vi "publish-measurements.vi"(5 "hash-format":string="{meas}:%d" caption="hash-format ({meas}:%d)", 7 "ttl":u64=30 caption="ttl (30s)", 8 "error in":errorcluster, 9 "measurement-list":string[](array[string]), 10 "period":u64, 11 "Redis in":refnum<class "Redis.lvclass">) -> (0 "error out":errorcluster, 2 "values":dbl[](array[numeric]), 3 "unix-time":u64)   [LabVIEW 2020, in "reporting-device.lvlib"]
uses:
  reporting-device.lvlib
  <userlib>/Zaphiro/GTools/Redis/Sources/Redis/Redis.lvclass
  <userlib>/Zaphiro/GTools/Redis/Sources/Redis/Redis.lvclass/Redis.ctl
  <userlib>/Zaphiro/GTools/Time/public/convert lv time to unix-scalar__ZGTools.vi
  <userlib>/Zaphiro/GTools/Redis/Sources/Redis/Connection/Send-command.vi
  <userlib>/Zaphiro/GTools/Redis/Sources/Redis/subVIs/LL_collect-response.vi
  <userlib>/Zaphiro/GTools/Time/time__ZGTools.lvlib
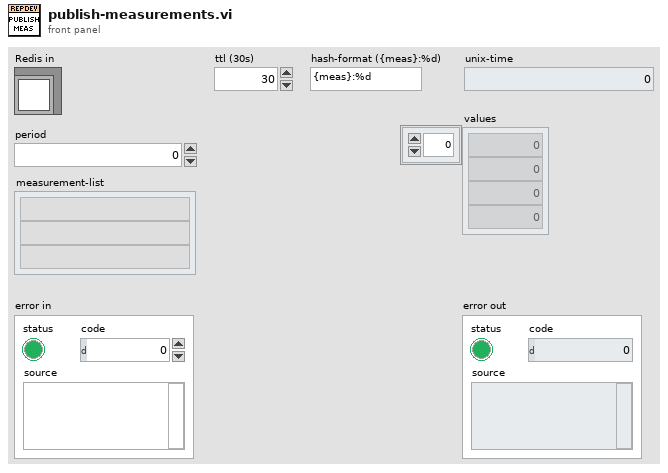
[diagram p1: front panel]
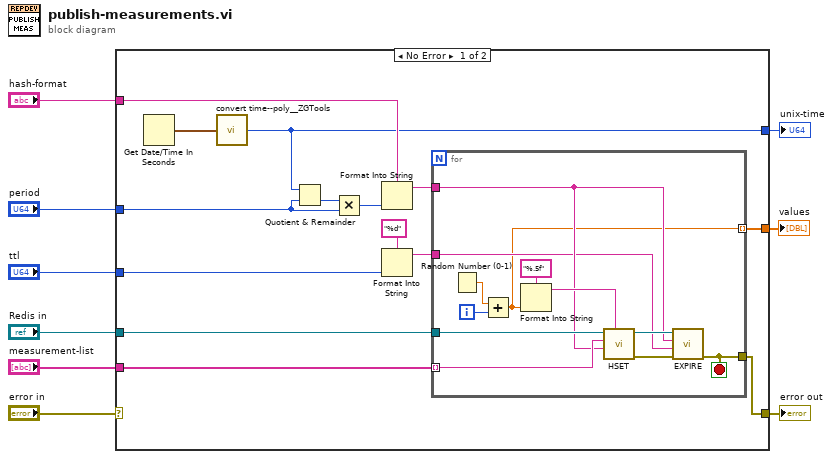
[diagram p0: block diagram]
diagram:
  n1 = case shown="No Error" "error in" {
    selector: "error in" -> [_ w36]
    tunnel: "measurement-list" -> [w23 _]
    tunnel: "period" -> [w22 _]
    tunnel: [w13 w36] -> w6
    tunnel: "Redis in" -> [w17 _]
    tunnel: "ttl" -> [w14 _]
    tunnel: "hash-format" -> [w12 _]
    tunnel: [w11 _] -> w2
    tunnel: [w10 _] -> w1
    frame No Error {
      n2 = Get Date/Time In Seconds() -> (seconds since 1Jan1904=w18:timestamp)
      n3 = call-poly <userlib>:"convert time--poly__ZGTools.vi"("labview-timestamp"=w18) -> ("unix-time"=w11:u64)  [unwired: 8 in]
      n4 = Quotient & Remainder(x=w11, y=w22) -> (floor(x/y)=w19:u64)  [unwired: 1 out]
      n5 = Multiply(x=w19, y=w22) -> (x*y=w20:u64)
      n6 = Format Into String(format string=w12, w20) -> (resulting string=w21:string)  [unwired: 2 in, 1 out]
      n7 = Format Into String(format string="%d" ("Seconds"), w14) -> (resulting string=w16:string)  [unwired: 2 in, 1 out]
      n8 = for {
        tunnel: w17 -> [w35]
        tunnel: w21 -> [w27]
        tunnel: w23 -> [w30] mode=indexing
        tunnel: w16 -> [w26]
        tunnel: [w25] -> w13
        tunnel: [w24] -> w10 mode=indexing
        i -> [w33]
        stop <- w25 stop-if-true
        n9 = Random Number (0-1)() -> (number: 0 to 1=w34:dbl)
        n10 = Add(x=w34, y=w33) -> (x+y=w24:dbl)
        n11 = Format Into String(format string="%.5f", w24) -> (resulting string=w32:string)  [unwired: 2 in, 1 out]
        n12 = call <userlib>:"HSET.vi"("Value"=w32, "Key"=w27, "Field"=w30, "Redis.lvclass in"=w35) -> ("error out"=w29:errorcluster, "Redis.lvclass out"=w28:refnum<class "Redis.lvclass">)  [unwired: 5 in, 1 out]
        n13 = call <userlib>:"EXPIRE.vi"("error in"=w29, "Seconds"=w26, "Key"=w27, "Redis.lvclass in"=w28) -> ("error out"=w25:errorcluster)  [unwired: 5 in, 2 out]
      }
    }
    frame Error {
    }
  }
  "error out" <- w6
  "unix-time" <- w2
  "values" <- w1
